vi "resetOutput.vi"(8 "error in (no error)":errorcluster, 11 "niDAQmxDO in":refnum<class "niDAQmxDO.lvclass">) -> (0 "error out":errorcluster, 3 "niDAQmxDO out":refnum<class "niDAQmxDO.lvclass">)   [LabVIEW 2011, in "Hardware.lvlib" / "Channels.lvlib" / "niDAQmxDO.lvclass"]
uses:
  niDAQmxDO.lvclass
  <vilib>/DAQmx/write.llb/DAQmx Write (Digital 2D U8 NChan NSamp).vi
  <vilib>/DAQmx/write.llb/DAQmx Write (Digital 1D Wfm NChan NSamp).vi
  <vilib>/DAQmx/create/channels.llb/DAQmx Create Channel (DO-Digital Output).vi
  <vilib>/DAQmx/configure/timing.llb/DAQmx Timing (Sample Clock).vi
  <vilib>/DAQmx/configure/trigger.llb/DAQmx Start Trigger (None).vi
  <vilib>/DAQmx/miscellaneous.llb/DAQmx Fill In Error Info.vi
  <vilib>/Waveform/DWDTOps.llb/DWDT Uncompress Digital.vi
  DigitalOutput.lvclass
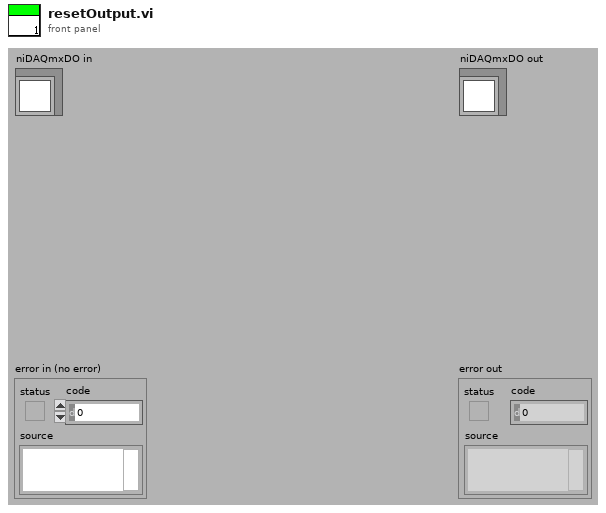
[diagram p1: front panel]
types:
  T1 = cluster{"Timestamps ms":dbl[], "Bitmap":bool[][]}
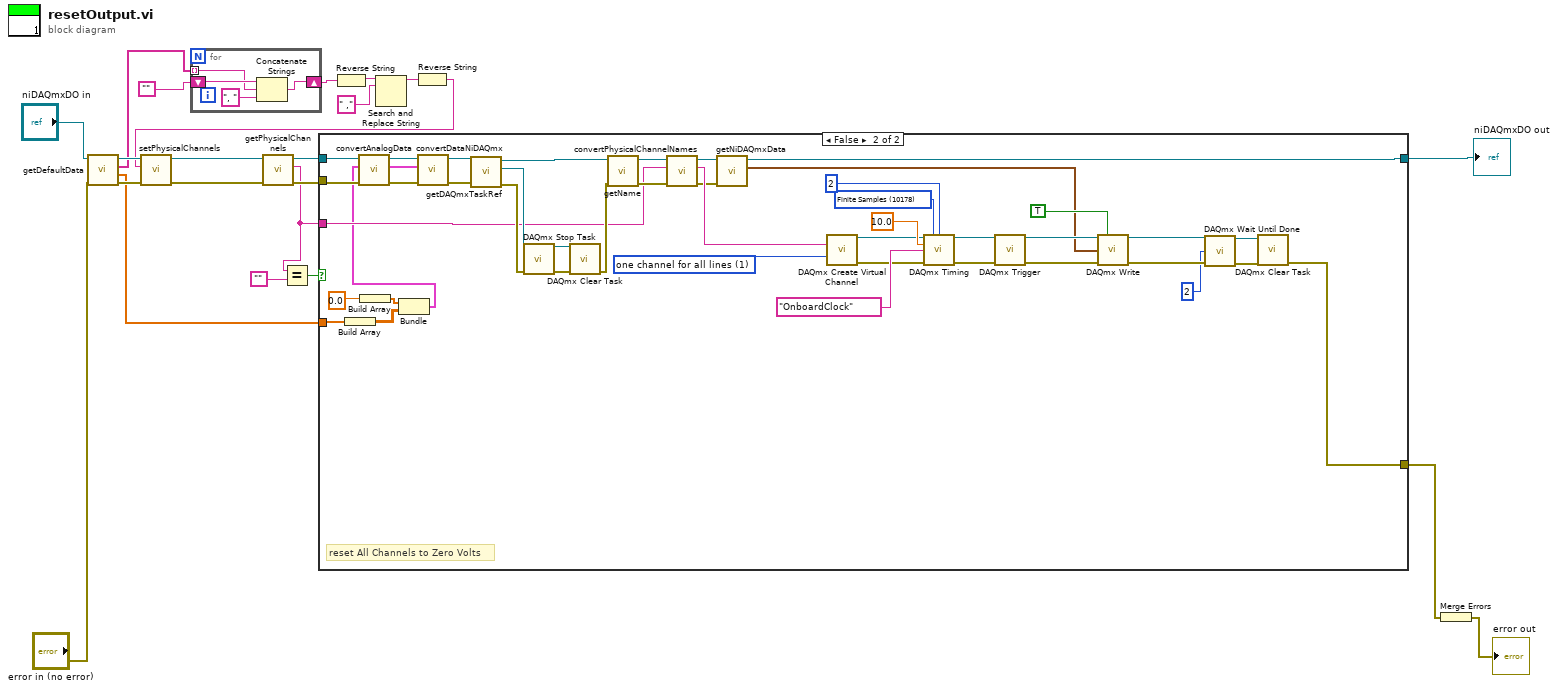
[diagram p0: block diagram]
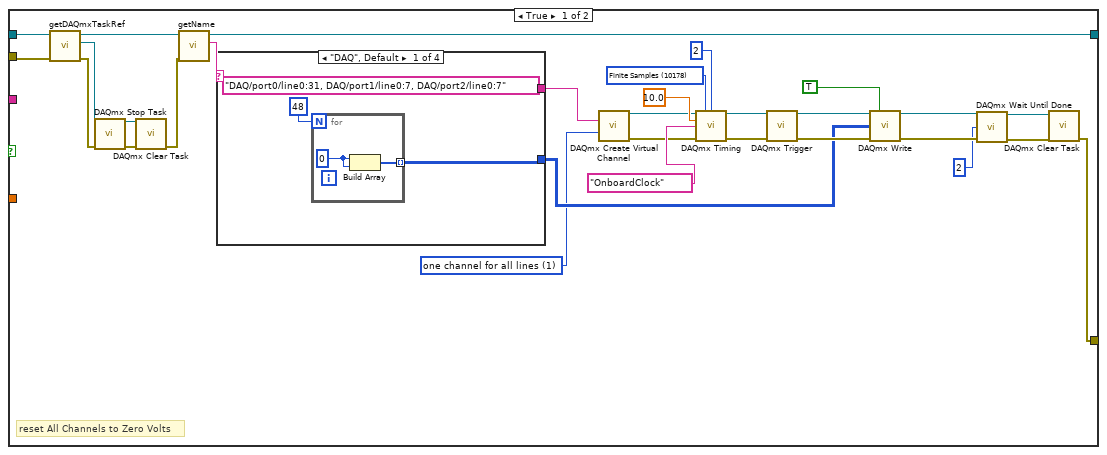
[diagram p2: hidden frame]
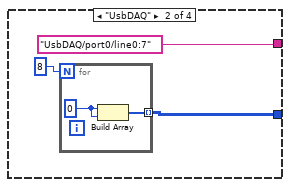
[diagram p3: hidden frame]
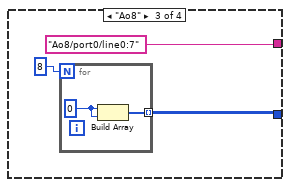
[diagram p4: hidden frame]
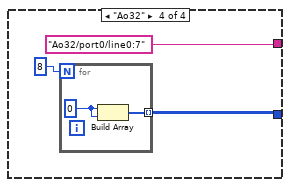
[diagram p5: hidden frame]
diagram:
  n1 = call "getDefaultData.vi"("error in (no error)"="error in (no error)", "DigitalOutput in"="niDAQmxDO in") -> ("error out"=w11:errorcluster, "calibratedValues"=w1:dbl[], "channel_addresses"=w3:string[], "DigitalOutput out"=w12:refnum<class "niDAQmxDO.lvclass">)  [unwired: 6 in]
  n2 = for {
    tunnel: w3 -> [w25] mode=indexing
    shift-right: [w23] -> w7
    shift-left: "" -> [w26]
    n3 = Concatenate Strings(w26, w25, ", ") -> (w23:string)
  }
  n4 = Reverse String(1:w7) -> (0:w6:string)
  n5 = Search and Replace String(input string=w6, search string=" ,") -> (result string=w4:string)  [unwired: 6 in, 3 out]
  n6 = Reverse String(1:w4) -> (0:w2:string)
  n7 = call-dynamic "setPhysicalChannels.vi"("error in (no error)"=w11, "Physical Channels"=w2, "DigitalOutput.lvclass in"=w12) -> ("error out"=w13:errorcluster, "DigitalOutput.lvclass out"=w14:refnum<class "niDAQmxDO.lvclass">)  [unwired: 7 in]
  n8 = call-dynamic "getPhysicalChannels.vi"("error in (no error)"=w13, "DigitalOutput.lvclass in"=w14) -> ("error out"=w16:errorcluster, "Physical Channels"=w15:string, "DigitalOutput.lvclass out"=w17:refnum<class "niDAQmxDO.lvclass">)  [unwired: 7 in]
  n9 = Equal?(x=w15, y="") -> (x = y?=w22:bool)
  n10 = case shown="False" w22 {
    tunnel: w15 -> [_ w94]
    tunnel: w16 -> [w34 w91]
    tunnel: [w38 w103] -> w20
    tunnel: w17 -> [w35 w92]
    tunnel: [w27 w77] -> w18
    tunnel: w1 -> [_ w90]
    frame True {
      w29 = 1 items=["one channel for each line", "one channel for all lines"] ("line grouping")
      w54 = 10178 items=["Finite Samples"=10178, "Continuous Samples"=10123, "Hardware Timed Single Point"=12522] ("sample mode")
      # "reset All Channels to Zero Volts"
      n11 = call "getDAQmxTaskRef.vi"("error in (no error)"=w34, "niDAQmxDO.lvclass in"=w35) -> ("error out"=w33:errorcluster, "DAQmx Task Ref"=w32:refnum<k21>, "niDAQmxDO.lvclass out"=w28:refnum<class "niDAQmxDO.lvclass">)  [unwired: 7 in]
      n12 = call <vilib>:"DAQmx Stop Task.vi"("task/channels in"=w32, "error in"=w33) -> ("task out"=w50:refnum<k21>, "error out"=w49:errorcluster)  [unwired: 12 in]
      n13 = call <vilib>:"DAQmx Clear Task.vi"("task in"=w50, "error in"=w49) -> ("error out"=w30:errorcluster)  [unwired: 13 in]
      n14 = call-dynamic "getName.vi"("error in (no error)"=w30, "DigitalOutput.lvclass in"=w28) -> ("name"=w31:string, "DigitalOutput.lvclass out"=w27:refnum<class "niDAQmxDO.lvclass">)  [unwired: 7 in, 1 out]
      n15 = case shown="\"DAQ\", Default" w31 {
        tunnel: ["DAQ/port0/line0:31, DAQ/port1/line0:7, DAQ/port2/line0:7" "UsbDAQ/port0/line0:7" "Ao8/port0/line0:7" "Ao32/port0/line0:7"] -> w48
        tunnel: [w59 w63 w68 w73] -> w36
        frame "DAQ", Default {
          n16 = for {
            N: 48 -> [_]
            tunnel: [w60] -> w59 mode=indexing
            w61 = u8 0
            n17 = Build Array(w61, w61) -> (w60:u8[])
          }
        }
        frame "UsbDAQ" {
          n18 = for {
            N: 8 -> [_]
            tunnel: [w65] -> w63 mode=indexing
            w66 = u8 0
            n19 = Build Array(w66, w66) -> (w65:u8[])
          }
        }
        frame "Ao8" {
          n20 = for {
            N: 8 -> [_]
            tunnel: [w70] -> w68 mode=indexing
            w71 = u8 0
            n21 = Build Array(w71, w71) -> (w70:u8[])
          }
        }
        frame "Ao32" {
          n22 = for {
            N: 8 -> [_]
            tunnel: [w75] -> w73 mode=indexing
            w76 = u8 0
            n23 = Build Array(w76, w76) -> (w75:u8[])
          }
        }
      }
      n24 = call-poly <vilib>:"DAQmx Create Virtual Channel.vi"("lines"=w48, "line grouping"=w29) -> ("task out"=w47:refnum<k21>, "error out"=w46:errorcluster)  [unwired: 12 in]
      n25 = call-poly <vilib>:"DAQmx Timing.vi"("task/channels in"=w47, "sample mode"=w54, "samples per channel"=2, "rate"=10.0, "source"=tag "OnboardClock", "error in"=w46) -> ("task out"=w52:refnum<k21>, "error out"=w51:errorcluster)  [unwired: 8 in]
      n26 = call-poly <vilib>:"DAQmx Trigger.vi"("task/channels in"=w52, "error in"=w51) -> ("task out"=w45:refnum<k21>, "error out"=w43:errorcluster)  [unwired: 12 in]
      n27 = call-poly <vilib>:"DAQmx Write.vi"("task/channels in"=w45, "auto start"=TRUE, "data"=w36, "error in"=w43) -> ("task out"=w42:refnum<k21>, "error out"=w41:errorcluster)  [unwired: 9 in, 1 out]
      n28 = call <vilib>:"DAQmx Wait Until Done.vi"("task/channels in"=w42, "timeout (sec)"=2, "error in"=w41) -> ("task out"=w40:refnum<k21>, "error out"=w39:errorcluster)  [unwired: 11 in]
      n29 = call <vilib>:"DAQmx Clear Task.vi"("task in"=w40, "error in"=w39) -> ("error out"=w38:errorcluster)  [unwired: 13 in]
    }
    frame False {
      w98 = 1 items=["one channel for each line", "one channel for all lines"] ("line grouping")
      w118 = 10178 items=["Finite Samples"=10178, "Continuous Samples"=10123, "Hardware Timed Single Point"=12522] ("sample mode")
      # "reset All Channels to Zero Volts"
      n30 = Build Array(w90) -> (w88:dbl[][])
      n31 = Build Array(0.0) -> (w87:dbl[])
      n32 = Bundle(w87, w88) -> (w86:cluster{dbl[], dbl[][]})  [unwired: 1 in]
      n33 = call "convertAnalogData.vi"("error in (no error)"=w91, "Data"=w86, "niDAQmxDO in"=w92) -> ("error out"=w85:errorcluster, "digitalData"=w82:T1, "niDAQmxDO out"=w84:refnum<class "niDAQmxDO.lvclass">)  [unwired: 6 in]
      n34 = call "convertDataNiDAQmx.vi"("error in (no error)"=w85, "Data"=w82, "niDAQmxDO in"=w84) -> ("error out"=w81:errorcluster, "niDAQmxDO out"=w83:refnum<class "niDAQmxDO.lvclass">)  [unwired: 7 in]
      n35 = call "getDAQmxTaskRef.vi"("error in (no error)"=w81, "niDAQmxDO.lvclass in"=w83) -> ("error out"=w101:errorcluster, "DAQmx Task Ref"=w100:refnum<k21>, "niDAQmxDO.lvclass out"=w97:refnum<class "niDAQmxDO.lvclass">)  [unwired: 7 in]
      n36 = call <vilib>:"DAQmx Stop Task.vi"("task/channels in"=w100, "error in"=w101) -> ("task out"=w114:refnum<k21>, "error out"=w113:errorcluster)  [unwired: 12 in]
      n37 = call <vilib>:"DAQmx Clear Task.vi"("task in"=w114, "error in"=w113) -> ("error out"=w99:errorcluster)  [unwired: 13 in]
      n38 = call-dynamic "getName.vi"("error in (no error)"=w99, "DigitalOutput.lvclass in"=w97) -> ("error out"=w95:errorcluster, "DigitalOutput.lvclass out"=w96:refnum<class "niDAQmxDO.lvclass">)  [unwired: 7 in, 1 out]
      n39 = call "convertPhysicalChannelNames.vi"("error in (no error)"=w95, "PhysicalChannels"=w94, "niDAQmxDO in"=w96) -> ("error out"=w79:errorcluster, "channel_names"=w93:string, "niDAQmxDO out"=w80:refnum<class "niDAQmxDO.lvclass">)  [unwired: 6 in]
      n40 = call "getNiDAQmxData.vi"("error in (no error)"=w79, "niDAQmxDO.lvclass in"=w80) -> ("NIDAQmx data format"=w78:digitalwaveform[], "niDAQmxDO.lvclass out"=w77:refnum<class "niDAQmxDO.lvclass">)  [unwired: 7 in, 1 out]
      n41 = call-poly <vilib>:"DAQmx Create Virtual Channel.vi"("lines"=w93, "line grouping"=w98) -> ("task out"=w112:refnum<k21>, "error out"=w111:errorcluster)  [unwired: 12 in]
      n42 = call-poly <vilib>:"DAQmx Timing.vi"("task/channels in"=w112, "sample mode"=w118, "samples per channel"=2, "rate"=10.0, "source"=tag "OnboardClock", "error in"=w111) -> ("task out"=w116:refnum<k21>, "error out"=w115:errorcluster)  [unwired: 8 in]
      n43 = call-poly <vilib>:"DAQmx Trigger.vi"("task/channels in"=w116, "error in"=w115) -> ("task out"=w110:refnum<k21>, "error out"=w108:errorcluster)  [unwired: 12 in]
      n44 = call-poly <vilib>:"DAQmx Write.vi"("task/channels in"=w110, "auto start"=TRUE, "data"=w78, "error in"=w108) -> ("task out"=w107:refnum<k21>, "error out"=w106:errorcluster)  [unwired: 9 in, 1 out]
      n45 = call <vilib>:"DAQmx Wait Until Done.vi"("task/channels in"=w107, "timeout (sec)"=2, "error in"=w106) -> ("task out"=w105:refnum<k21>, "error out"=w104:errorcluster)  [unwired: 11 in]
      n46 = call <vilib>:"DAQmx Clear Task.vi"("task in"=w105, "error in"=w104) -> ("error out"=w103:errorcluster)  [unwired: 13 in]
    }
  }
  "niDAQmxDO out" <- w18
  n47 = Merge Errors(w20) -> (→"error out":errorcluster)
